vi "svx_Polar_Get_Data.vi"(0 "polar plot":T1, 5 "error in":errorcluster) -> (14 "polar plot out":T1, 15 "magnitude":dbl[](array[numeric]), 16 "phase":dbl[](array[numeric]), 17 "time/rev/RPM":dbl[](array[numeric]), 18 "attribute":variant, 19 "error out":errorcluster)   [LabVIEW 2017, in "SVX Polar Plot.xctl"]
uses:
  <vilib>/addons/_XControls/Polar Plot/SVX Polar Plot.xctl
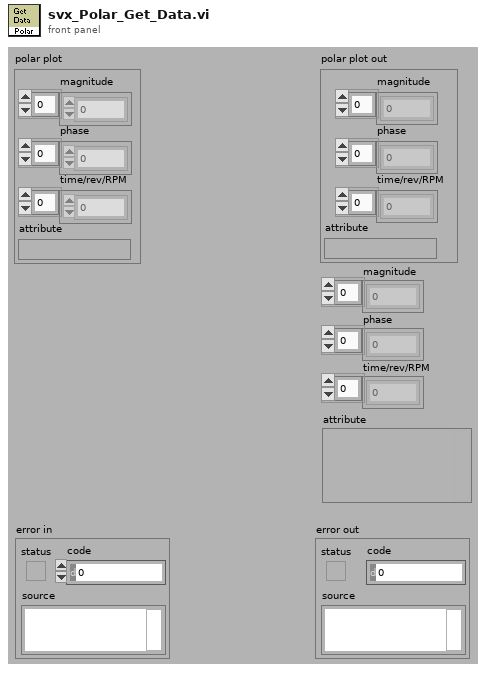
[diagram p1: front panel]
types:
  T1 = cluster{"magnitude":dbl[], "phase":dbl[], "time/rev/RPM":dbl[], "attribute":variant}
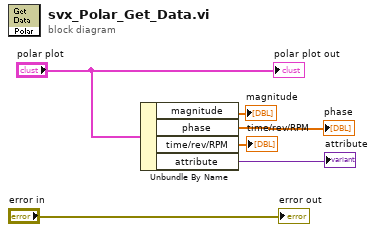
[diagram p0: block diagram]
diagram:
  n1 = Unbundle By Name("polar plot") -> ("magnitude"=→"magnitude":dbl[], "phase"=→"phase":dbl[], "time/rev/RPM"=→"time/rev/RPM":dbl[], "attribute"=→"attribute":variant)
  "error out" <- "error in"
  "polar plot out" <- "polar plot"
